vi "DIAdem Parameter File.vi"(4 "error in (no error)":errorcluster, 6 "Parameter":string, 7 "File Directory":path) -> (0 "error out":errorcluster, 3 "Parameter File":path)   [LabVIEW 2017]
doc: "This VI creates a temporary diadem readable parameter file."
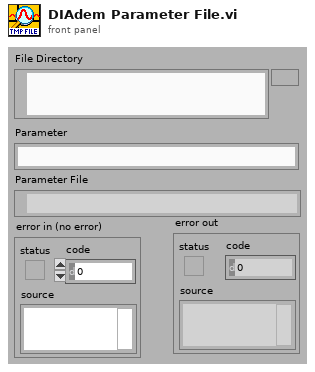
[diagram p1: front panel]
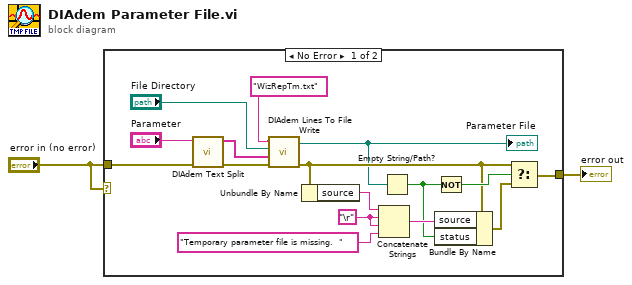
[diagram p0: block diagram]
diagram:
  n1 = case shown="No Error" "error in (no error)" {
    tunnel: "error in (no error)" -> [w6 w19]
    tunnel: [w14 w19] -> w1
    frame No Error {
      w18 = "\r"
      n2 = call <vilib>:"DIAdem Text Split.vi"("error in (no error)"=w6, "Full Input Text"="Parameter") -> ("error out"=w5:errorcluster, "Output Strings"=w3:string[])  [unwired: 4 in]
      n3 = call <vilib>:"DIAdem Lines To File Write.vi"("error in (no error)"=w5, "File Entries"=w3, "File Path"="File Directory", "File Name"="WizRepTm.txt" ("VBS Sequence Name")) -> ("error out"=w10:errorcluster, "Result File Path"=w7:path)  [unwired: 2 in]
      "Parameter File" <- w7
      n4 = Unbundle By Name(w10) -> ("source"=w15:string)
      n5 = Concatenate Strings(w15, w18, w18, "Temporary parameter file is missing.  " ("source")) -> (w17:string)
      n6 = Empty String/Path?(string/path=w7) -> (empty?=w11:bool)
      n7 = Bundle By Name(cluster=w10, "source"=w17, "status"=w11) -> (w12:errorcluster)
      n8 = Not(x=w11) -> (.not. x?=w13:bool)
      n9 = Select(t=w10, s=w13, f=w12) -> (s? t:f=w14:errorcluster)
    }
    frame Error {
    }
  }
  "error out" <- w1
